vi "Lift.vi"() -> ()   [LabVIEW 2014]
uses:
  <vilib>/NXT/Subs/MotorOutput.ctl
  <vilib>/Analysis/1siggen.llb/Ramp Pattern by Samples.vi
  <vilib>/NXT/Dual Mode Library/Motors/ResetMotor.vi
  <vilib>/NXT/Dual Mode Library/Motors/Rotation.vi
  <vilib>/NXT/Dual Mode Library/Motors/MotorOn.vi
  <vilib>/Analysis/NI_AALBase.lvlib
panel:
  in  "UP":bool
  in  "Down":bool
  in  "samples":i32=500
  in  "End":sgl=150.0 format="%#_13g"
  in  "End":sgl=60.0 format="%#_13g"
  in  "Start":sgl=15.0 format="%#_13g"
  in  "Start":sgl format="%#_13g"
  in  "Gain":sgl=6.0 format="%#_13g"
  in  "Gain":sgl=4.0 format="%#_13g"
  in  "Front Lift":i32(slide) scale=0.0..100.0
  in  "stop":bool=TRUE
  in  "Back Lift":i32(slide) scale=0.0..100.0
  # "Front"
  # "Back"
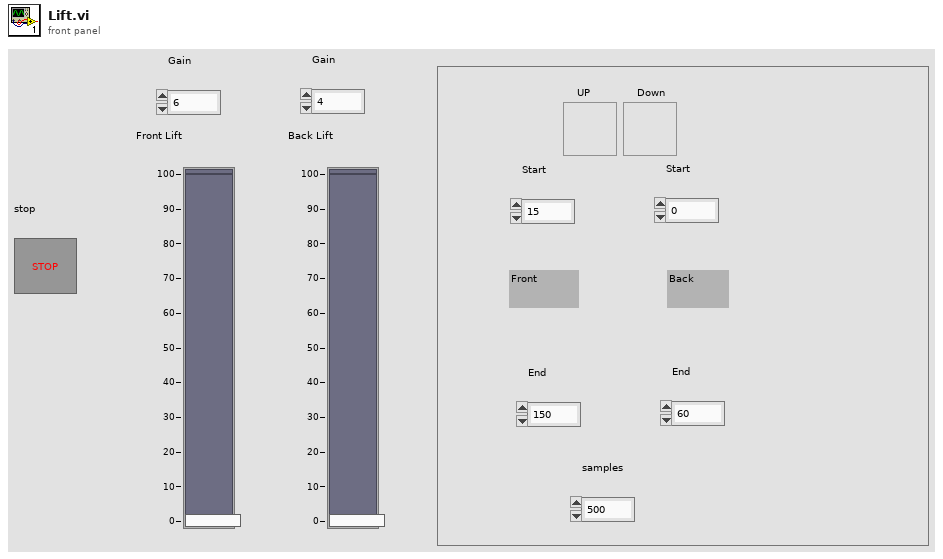
[diagram p1: front panel]
types:
  T1 = typedef "MotorOutput.ctl" = u8
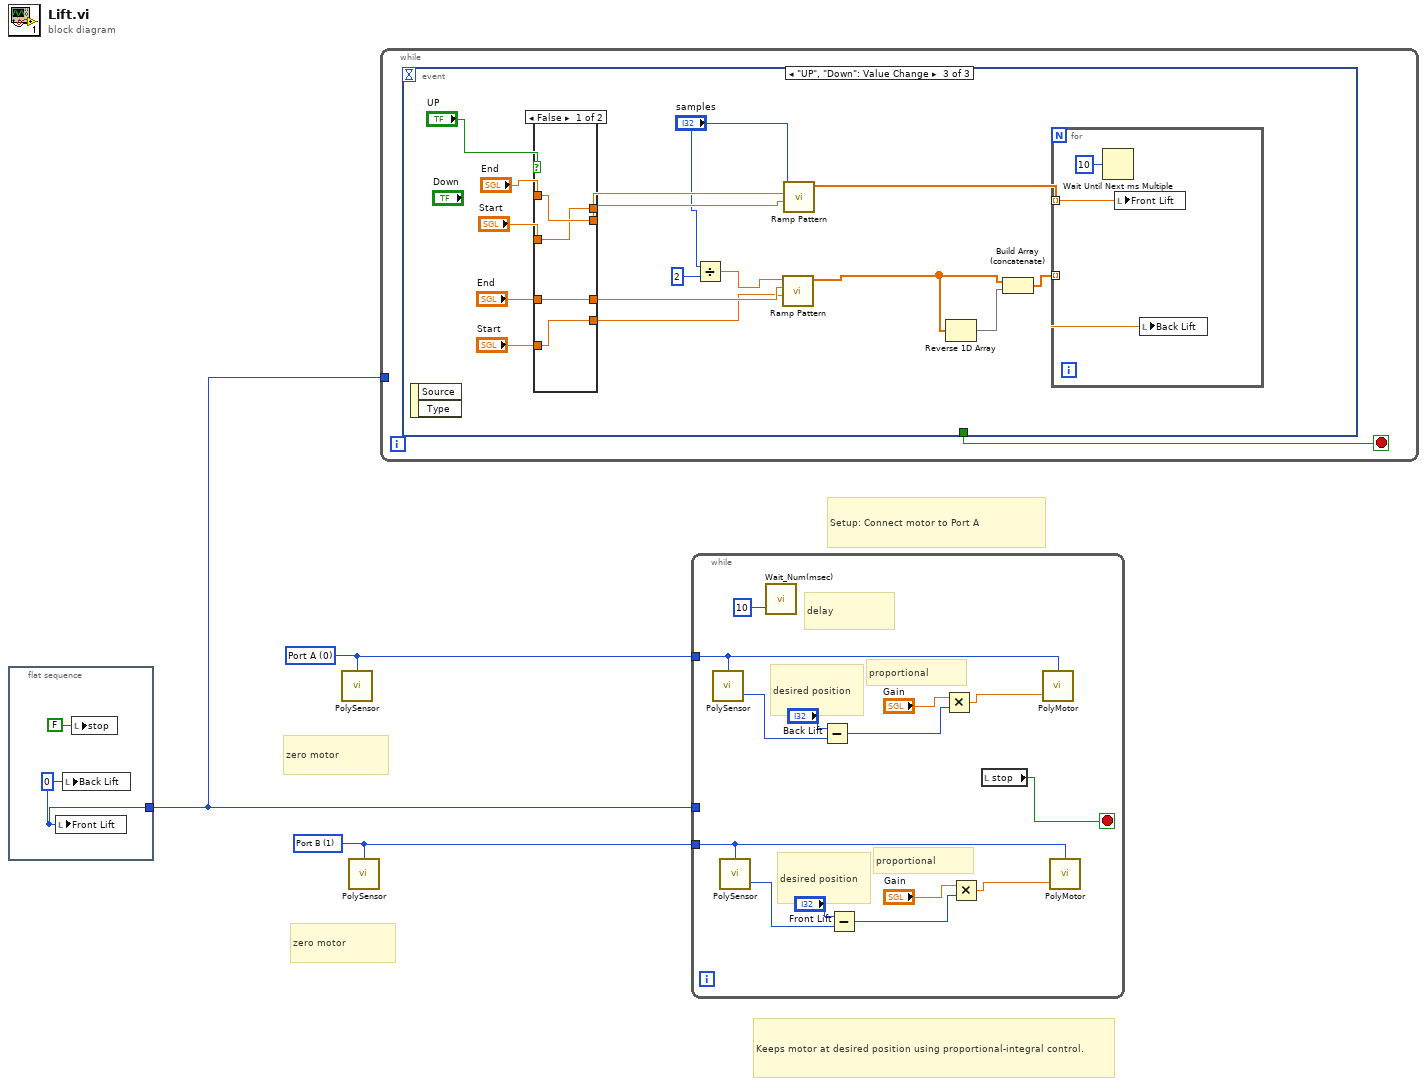
[diagram p0: block diagram]
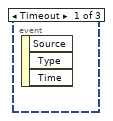
[diagram p2: hidden frame]
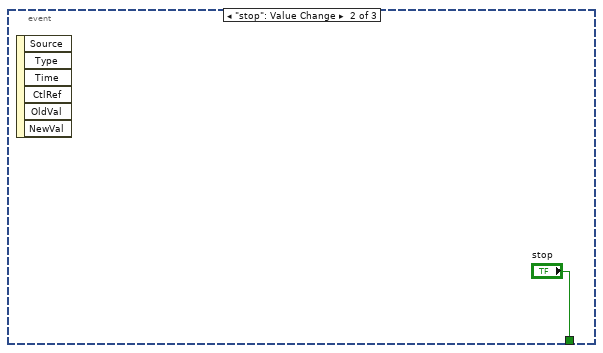
[diagram p3: hidden frame]
diagram:
  w2 = T1 1 items=["Port A"=0, "Port B"=1, "Port C"=2, "Ports A & B"=4, "Ports A & C"=5, "Ports B & C"=6, "All Ports"=3] ("Port (All Ports)")
  w3 = T1 0 items=["Port A"=0, "Port B"=1, "Port C"=2, "Ports A & B"=4, "Ports A & C"=5, "Ports B & C"=6, "All Ports"=3] ("Port (All Ports)")
  # "zero motor"
  # "zero motor"
  # "Keeps motor at desired position using proportional-integral control."
  # "Setup: Connect motor to Port A"
  n1 = flat-sequence {
    tunnel: [w5] -> w1
    frame #0 {
      w5 = 0 ("Back Lift")
      n2 = local write "Front Lift"(w5) -> ()
      n3 = local write "Back Lift"(w5) -> ()
      n4 = local write "stop"(FALSE ("stop")) -> ()
    }
  }
  n5 = call-poly <vilib>:"PolySensor.vi"("Port (All Ports)"=w3) -> ()  [unwired: 1 in, 3 out]
  n6 = call-poly <vilib>:"PolySensor.vi"("Port (All Ports)"=w2) -> ()  [unwired: 1 in, 3 out]
  n7 = while {
    tunnel: w1 -> [_]
    stop <- w6 stop-if-true
    n8 = event shown="[2] \"UP\", \"Down\": Value Change" {
      selector: _ -> [_ _ _]
      dyn-events: _ -> [_ _ _]
      timeout: _ -> [_ _ _]
      tunnel: [_ "stop" _] -> w6
      event Timeout {
        n9 = event-data() -> ()  [unwired: 1 in, 3 out]
      }
      event "stop": Value Change {
        n10 = event-data() -> ()  [unwired: 1 in, 6 out]
      }
      event "UP", "Down": Value Change {
        n11 = event-data() -> ()  [unwired: 1 in, 2 out]
        n12 = case shown="False" "UP" {
          tunnel: "End" -> [w27 w31]
          tunnel: [w26 w31] -> w20
          tunnel: [w27 w30] -> w19
          tunnel: "Start" -> [w26 w30]
          tunnel: [w24 w29] -> w17
          tunnel: "End" -> [w24 w29]
          tunnel: [w25 w28] -> w15
          tunnel: "Start" -> [w25 w28]
          frame False {
          }
          frame True {
          }
        }
        n13 = Divide(x="samples", y=2) -> (x/y=w12:dbl)
        n14 = call-poly <vilib>:"Ramp Pattern.vi"("start"=w15, "end"=w17, "samples"=w12) -> ("Ramp Pattern"=w9:dbl[])  [unwired: 7 in, 1 out]
        n15 = call-poly <vilib>:"Ramp Pattern.vi"("start"=w19, "end"=w20, "samples"="samples") -> ("Ramp Pattern"=w23:dbl[])  [unwired: 7 in, 1 out]
        n16 = Reverse 1D Array(array=w9) -> (reversed array=w8:dbl[])
        n17 = Build Array (concatenate)(w9, w8) -> (w10:dbl[])
        n18 = for {
          tunnel: w23 -> [w33] mode=indexing
          tunnel: w10 -> [w32] mode=indexing
          n19 = Wait Until Next ms Multiple(millisecond multiple=u32 10) -> ()  [unwired: 1 out]
          n20 = local write "Front Lift"(w33) -> ()
          n21 = local write "Back Lift"(w32) -> ()
        }
      }
    }
  }
  n22 = while {
    tunnel: w3 -> [w43]
    tunnel: w2 -> [w42]
    tunnel: w1 -> [_]
    stop <- w35 stop-if-true
    # "proportional"
    # "desired position"
    # "proportional"
    # "desired position"
    # "delay"
    n23 = call-poly <vilib>:"PolySensor.vi"("Port (Port A)"=w43) -> ("Angle of Rotation"=w45:i32)  [unwired: 1 in, 2 out]
    n24 = call-poly <vilib>:"PolySensor.vi"("Port (Port A)"=w42) -> ("Angle of Rotation"=w41:i32)  [unwired: 1 in, 2 out]
    n25 = call <vilib>:"Wait_Num(msec).vi"("Time (100 msec)"=u32 10 ("milliseconds to wait")) -> ()  [unwired: 3 in, 1 out]
    n26 = Subtract(x="Back Lift", y=w45) -> (x-y=w46:i32)
    n27 = Subtract(x="Front Lift", y=w41) -> (x-y=w40:i32)
    n28 = Multiply(x="Gain", y=w46) -> (x*y=w37:sgl)
    n29 = Multiply(x="Gain", y=w40) -> (x*y=w36:sgl)
    n30 = local read "stop"() -> (w35:bool)
    n31 = call-poly <vilib>:"PolyMotor.vi"("Power (75)"=w37, "Output Port (All Ports)"=w43) -> ()  [unwired: 1 in, 2 out]
    n32 = call-poly <vilib>:"PolyMotor.vi"("Power (75)"=w36, "Output Port (All Ports)"=w42) -> ()  [unwired: 1 in, 2 out]
  }
